vi "toggle.vi"(11 "In":bool) -> (3 "Out":bool)   [LabVIEW 2013]
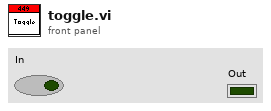
[diagram p1: front panel]
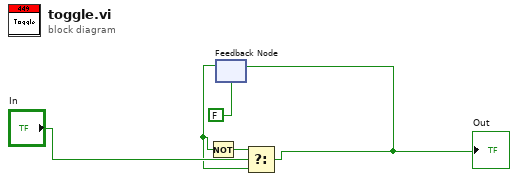
[diagram p0: block diagram]
diagram:
  n1 = feedback #1(FALSE) -> (w1:bool)
  n2 = Not(x=w1) -> (.not. x?=w2:bool)
  n3 = Select(t=w2, s="In", f=w1) -> (s? t:f=w3:bool)
  "Out" <- w3
  n4 = feedback-in #1(w3) -> ()
